vi "Intake Rollers.vi"   [LabVIEW 2014]
uses:
  Begin/Global RefNums.vi
  Begin/Global Variables.vi
  <vilib>/Rock Robotics/WPI/Solenoid/Deprecated/WPI_SolenoidSetBool.vi
types:
  T1 = typedef "WPI_MotorControlDeviceRef.ctl" = cluster{"DeviceStatus":errorcluster, "Type":T2, "PWM":cluster{"Controller":T3, "PWM Channel":T4, "DeadBand":T5}, "CAN":cluster{"Device Number":u8, "Control Mode":T6, "Semaphore":T7, "Max Vout":dbl, "TalonSRX Control Mode":T8}, "Invert":bool, "TransformRef":T9, "InvTransformRef":T9}
  T2 = typedef "WPI_MotorControlType.ctl" = enum16{"PWM", "CAN", "CANTalonSRX"}
  T3 = typedef "FPGA_TypedefDigitalModule.ctl" = enum16{"Controller 1"}
  T4 = typedef "FPGA_DIOPWMChannel.ctl" = enum8{"PWM 0", "PWM 1", "PWM 2", "PWM 3", "PWM 4", "PWM 5", "PWM 6", "PWM 7", "PWM 8", "PWM 9", "PWM MXP 0", "PWM MXP 1", "PWM MXP 2", "PWM MXP 3", "PWM MXP 4", "PWM MXP 5", "PWM MXP 6", "PWM MXP 7", "PWM MXP 8", "PWM MXP 9", "Invalid"}
  T5 = typedef "WPI_PWMDeadband.ctl" = cluster{"Name":string, "maxPositivePwm":i32, "minPositivePwm":i32, "centerPwm":i32, "maxNegativePwm":i32, "minNegativePwm":i32, "angularRange":u16}
  T6 = typedef "WPI_CANJaguar_ControlMode.ctl" = enum8{"Percent VBus", "Current", "Speed", "Position", "Voltage"}
  T7 = typedef "Semaphore RefNum" = refnum<k1>
  T8 = typedef "WPI_CANTalonSRX_APIControlMode.ctl" = enum8{"Percent VBus", "Speed", "Position", "Slave", "Unchanged / Invalid"}
  T9 = typedef "WPI_PWMTransform_ConPane.ctl" = refnum<vi>
  T10 = typedef "WPI_SolenoidDevRef.ctl" = cluster{"DevStatus":errorcluster, "Pneumatics Control Module":u8, "Forward Solenoid Channel":T11, "Reverse Solenoid Channel":T11}
  T11 = typedef "WPI_SolenoidChannel.ctl" = enum8{"Solenoid 0", "Solenoid 1", "Solenoid 2", "Solenoid 3", "Solenoid 4", "Solenoid 5", "Solenoid 6", "Solenoid 7", "Invalid"}
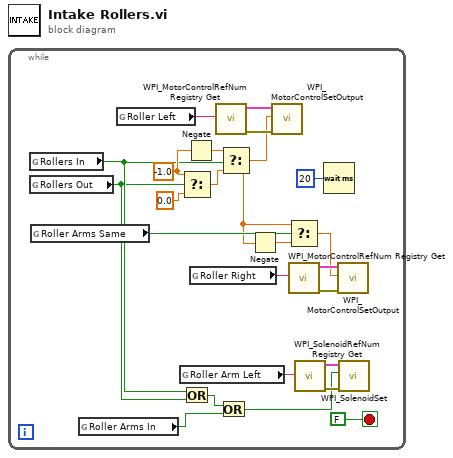
[diagram p0: block diagram]
diagram:
  n1 = while {
    stop <- FALSE stop-if-true
    w15 = -1.0 ("t")
    n2 = global read "Global Variables.vi" "Rollers In"() -> (w14:bool)
    n3 = global read "Global Variables.vi" "Rollers Out"() -> (w13:bool)
    n4 = global read "Global Variables.vi" "Roller Arms Same"() -> (w4:bool)
    n5 = global read "Global Variables.vi" "Roller Arms In"() -> (w11:bool)
    n6 = global read "Global RefNums.vi" "Roller Left"() -> (w22:string)
    n7 = global read "Global RefNums.vi" "Roller Arm Left"() -> (w8:string)
    n8 = Select(t=w15, s=w13, f=0.0) -> (s? t:f=w18:dbl)
    n9 = Or(x=w14, y=w13) -> (x .or. y?=w12:bool)
    n10 = Negate(x=w15) -> (-x=w16:dbl)
    n11 = global read "Global RefNums.vi" "Roller Right"() -> (w21:string)
    n12 = call <vilib>:"WPI_MotorControlRefNum Registry Get.vi"("refnum name"=w22) -> ("error out"=w24:errorcluster, "MotorControlDevRef"=w23:T1)  [unwired: 9 in]
    n13 = Or(x=w12, y=w11) -> (x .or. y?=w7:bool)
    n14 = Select(t=w16, s=w14, f=w18) -> (s? t:f=w2:dbl)
    n15 = Negate(x=w2) -> (-x=w1:dbl)
    n16 = call <vilib>:"WPI_MotorControlSetOutput.vi"("error in (no error)"=w24, "Output"=w2, "MotorControlDevRef"=w23) -> ()  [unwired: 6 in, 3 out]
    n17 = Select(t=w2, s=w4, f=w1) -> (s? t:f=w3:dbl)
    n18 = call <vilib>:"WPI_MotorControlRefNum Registry Get.vi"("refnum name"=w21) -> ("error out"=w19:errorcluster, "MotorControlDevRef"=w20:T1)  [unwired: 9 in]
    n19 = call <vilib>:"WPI_SolenoidRefNum Registry Get.vi"("refnum name"=w8) -> ("error out"=w10:errorcluster, "SolenoidDevRef"=w9:T10)  [unwired: 9 in]
    n20 = Wait (ms)(milliseconds to wait=u32 20) -> ()  [unwired: 1 out]
    n21 = call <vilib>:"WPI_MotorControlSetOutput.vi"("error in (no error)"=w19, "Output"=w3, "MotorControlDevRef"=w20) -> ()  [unwired: 6 in, 3 out]
    n22 = call-poly <vilib>:"WPI_SolenoidSet.vi"("error in (no error)"=w10, "Value"=w7, "SolenoidDevRef"=w9) -> ()  [unwired: 7 in, 2 out]
  }
